vi "Initialize.vi"(8 "error in (no error)":errorcluster, 10 "DeviceName":string, 11 "FakePressureController in":refnum<class "PXIDigitizer.lvclass">) -> (0 "error out":errorcluster, 1 "new command(s)":string, 2 "DeviceName":string, 3 "FakePressureController out":refnum<class "PXIDigitizer.lvclass">)   [LabVIEW 2011, in "PXIDigitizer.lvclass"]
uses:
  PXIDigitizer.lvclass
  settings_TypDef.ctl
  numericVariable_TypeDef.ctl
  OnOffTypeDef.ctl
  channelenabled_TypDef.ctl
  coupling_Enum_TypDef.ctl
  impedance_Enum_TypDEf.ctl
  TriggerSettings_TypDef.ctl
  Polarity_TypDEf.ctl
  TVEvent_TypDef.ctl
  coupling_TypDef.ctl
  positive_negatice2_typDef.ctl
  TriggerSource_TypDef.ctl
  triggerwindowmode2_TypDef.ctl
  SignalFormat_TypDef.ctl
  mode_TypDef.ctl
  Trigger.DigitalSource_TypDEf.ctl
  horizontal_TypDef.ctl
  methodCluster_TypDEf.ctl
  method_TypDef.ctl
  LinkedChannelsCluster_TypDef.ctl
  channels_TypDef.ctl
  BaseDriver/BaseDriver.lvclass
  PXIDigitizer.lvclass/PXIDigitizer.ctl
panel:
  out "data":T1={"resourcename"="", "timeout"={"Value"=0.0, "Min"=0.0, "Max"=0.0, "StepSize"=0.0, "Tolerance"=0.0, "valueactual"=0.0}, "LocalSavingPath"=path "", "Save"=enum."off", "probeattenuation"={"Channel0"={"Value"=0.0, "Min"=0.0, "Max"=0.0, "StepSize"=0.0, "Tolerance"=0.0, "valueactual"=0.0}, "Channel1"={"Value"=0.0, "Min"=0.0, "Max"=0.0, "StepSize"=0.0, "Tolerance"=0.0, "valueactual"=0.0}, "Channel2"={"Value"=0.0, "Min"=0.0, "Max"=0.0, "StepSize"=0.0, "Tolerance"=0.0, "valueactual"=0.0}, "Channel3"={"Value"=0.0, "Min"=0.0, "Max"=0.0, "StepSize"=0.0, "Tolerance"=0.0, "valueactual"=0.0}, "Channel4"={"Value"=0.0, "Min"=0.0, "Max"=0.0, "StepSize"=0.0, "Tolerance"=0.0, "valueactual"=0.0}, "Channel5"={"Value"=0.0, "Min"=0.0, "Max"=0.0, "StepSize"=0.0, "Tolerance"=0.0, "valueactual"=0.0}, "Channel6"={"Value"=0.0, "Min"=0.0, "Max"=0.0, "StepSize"=0.0, "Tolerance"=0.0, "valueactual"=0.0}, "Channel7"={"Value"=0.0, "Min"=0.0, "Max"=0.0, "StepSize"=0.0, "Tolerance"=0.0, "valueactual"=0.0}}, "channelenabled"={"Channel0"=enum."off", "Channel1"=enum."off", "Channel2"=enum."off", "Channel3"=enum."off", "Channel4"=enum."off", "Channel5"=enum."off", "Channel6"=enum."off", "Channel7"=enum."off"}, "coupling"={"Channel0"=enum."AC", "Channel1"=enum."AC", "Channel2"=enum."AC", "Channel3"=enum."AC", "Channel4"=enum."AC", "Channel5"=enum."AC", "Channel6"=enum."AC", "Channel7"=enum."AC"}, "impedance"={"Channel0"=enum."1 mega ohm", "Channel1"=enum."1 mega ohm", "Channel2"=enum."1 mega ohm", "Channel3"=enum."1 mega ohm", "Channel4"=enum."1 mega ohm", "Channel5"=enum."1 mega ohm", "Channel6"=enum."1 mega ohm", "Channel7"=enum."1 mega ohm"}, "Trigger"={"DC Restore"=enum."off", "Polarity"=enum."Negative", "TV Event"=enum."Field 1", "Coupling"=enum."AC", "Slope"=enum."Negative", "AnalogSource"=enum."Channel 0", "Window Mode"=enum."Entering", "Low Level"=0.0, "High Level"=0.0, "Hysteresis"=0.0, "Delay"=0.0, "Holdoff"=0.0, "Signal Format"=enum."M-NTSC", "Mode"=enum."Immediate", "Line Number"=0, "DigitalSource"=enum."RTSI 0"}, "Horizontal"={"min sample rate"=10000000.0, "min record length"=1000, "actual record length"=1000, "actual sample rate"=10000000.0, "Enforce Realtime"=enum."off"}, "Names"={"Channel0"="", "Channel1"="", "Channel2"="", "Channel3"="", "Channel4"="", "Channel5"="", "Channel6"="", "Channel7"=""}, "verticalrange"={"Channel0"={"Value"=0.0, "Min"=0.0, "Max"=0.0, "StepSize"=0.0, "Tolerance"=0.0, "valueactual"=0.0}, "Channel1"={"Value"=0.0, "Min"=0.0, "Max"=0.0, "StepSize"=0.0, "Tolerance"=0.0, "valueactual"=0.0}, "Channel2"={"Value"=0.0, "Min"=0.0, "Max"=0.0, "StepSize"=0.0, "Tolerance"=0.0, "valueactual"=0.0}, "Channel3"={"Value"=0.0, "Min"=0.0, "Max"=0.0, "StepSize"=0.0, "Tolerance"=0.0, "valueactual"=0.0}, "Channel4"={"Value"=0.0, "Min"=0.0, "Max"=0.0, "StepSize"=0.0, "Tolerance"=0.0, "valueactual"=0.0}, "Channel5"={"Value"=0.0, "Min"=0.0, "Max"=0.0, "StepSize"=0.0, "Tolerance"=0.0, "valueactual"=0.0}, "Channel6"={"Value"=0.0, "Min"=0.0, "Max"=0.0, "StepSize"=0.0, "Tolerance"=0.0, "valueactual"=0.0}, "Channel7"={"Value"=0.0, "Min"=0.0, "Max"=0.0, "StepSize"=0.0, "Tolerance"=0.0, "valueactual"=0.0}}, "offset"={"Channel0"={"Value"=0.0, "Min"=0.0, "Max"=0.0, "StepSize"=0.0, "Tolerance"=0.0, "valueactual"=0.0}, "Channel1"={"Value"=0.0, "Min"=0.0, "Max"=0.0, "StepSize"=0.0, "Tolerance"=0.0, "valueactual"=0.0}, "Channel2"={"Value"=0.0, "Min"=0.0, "Max"=0.0, "StepSize"=0.0, "Tolerance"=0.0, "valueactual"=0.0}, "Channel3"={"Value"=0.0, "Min"=0.0, "Max"=0.0, "StepSize"=0.0, "Tolerance"=0.0, "valueactual"=0.0}, "Channel4"={"Value"=0.0, "Min"=0.0, "Max"=0.0, "StepSize"=0.0, "Tolerance"=0.0, "valueactual"=0.0}, "Channel5"={"Value"=0.0, "Min"=0.0, "Max"=0.0, "StepSize"=0.0, "Tolerance"=0.0, "valueactual"=0.0}, "Channel6"={"Value"=0.0, "Min"=0.0, "Max"=0.0, "StepSize"=0.0, "Tolerance"=0.0, "valueactual"=0.0}, "Channel7"={"Value"=0.0, "Min"=0.0, "Max"=0.0, "StepSize"=0.0, "Tolerance"=0.0, "valueactual"=0.0}}, "Number of channels"=0.0, "Method"={"Analysis1"=enum."max", "Analysis2"=enum."max", "Analysis3"=enum."max", "Analysis4"=enum."max", "Analysis5"=enum."max", "Analysis6"=enum."max", "Analysis7"=enum."max", "Analysis8"=enum."max", "Analysis9"=enum."max", "Analysis10"=enum."max"}, "LinkedChannel"={"Analysis1"=enum."Channel0", "Analysis2"=enum."Channel0", "Analysis3"=enum."Channel0", "Analysis4"=enum."Channel0", "Analysis5"=enum."Channel0", "Analysis6"=enum."Channel0", "Analysis7"=enum."Channel0", "Analysis8"=enum."Channel0", "Analysis9"=enum."Channel0", "Analysis10"=enum."Channel0"}} {"Horizontal"."actual sample rate" format="%.2p"; "Horizontal"."min sample rate" step=1000000.0 format="%.2p"; "Trigger"."Delay" format="%#_12e"; "Trigger"."Holdoff" format="%#_12e"}
  out "Settings.resourcename":string
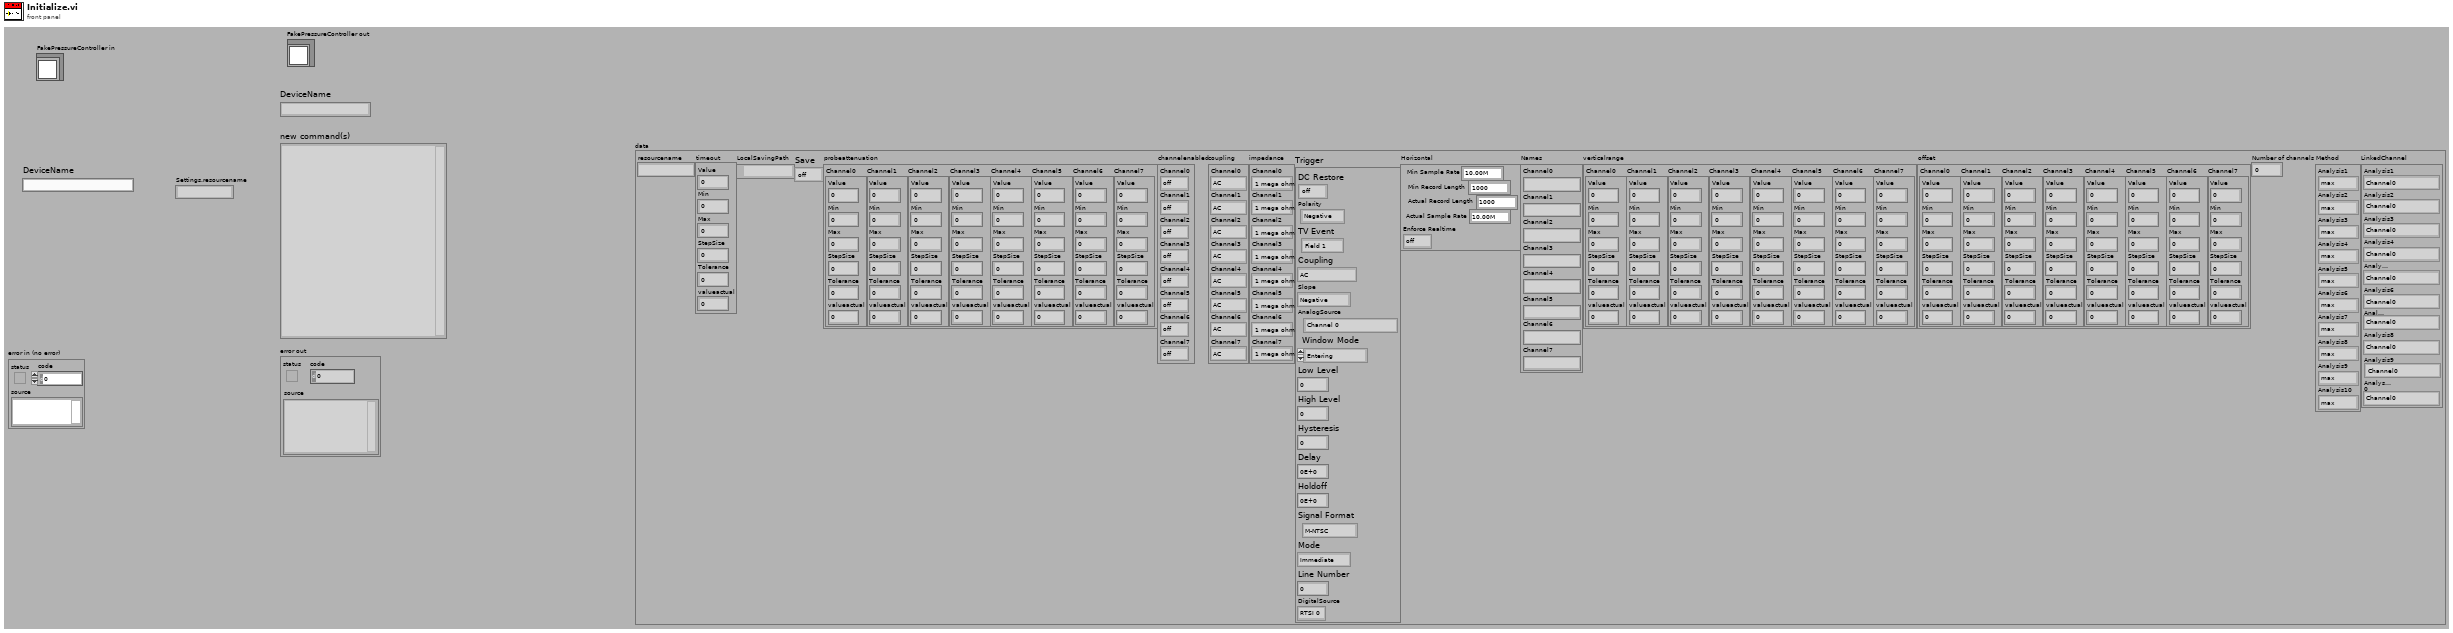
[diagram p1: front panel]
types:
  T1 = typedef "PXIDigitizer.lvclass/settings_TypDef.ctl" = cluster{"resourcename":string, "timeout":T2, "LocalSavingPath":path, "Save":T3, "probeattenuation":cluster{"Channel0":T2, "Channel1":T2, "Channel2":T2, "Channel3":T2, "Channel4":T2, "Channel5":T2, "Channel6":T2, "Channel7":T2}, "channelenabled":T4, "coupling":cluster{"Channel0":T5, "Channel1":T5, "Channel2":T5, "Channel3":T5, "Channel4":T5, "Channel5":T5, "Channel6":T5, "Channel7":T5}, "impedance":cluster{"Channel0":T6, "Channel1":T6, "Channel2":T6, "Channel3":T6, "Channel4":T6, "Channel5":T6, "Channel6":T6, "Channel7":T6}, "Trigger":T7, "Horizontal":T17, "Names":cluster{"Channel0":string, "Channel1":string, "Channel2":string, "Channel3":string, "Channel4":string, "Channel5":string, "Channel6":string, "Channel7":string}, "verticalrange":cluster{"Channel0":T2, "Channel1":T2, "Channel2":T2, "Channel3":T2, "Channel4":T2, "Channel5":T2, "Channel6":T2, "Channel7":T2}, "offset":cluster{"Channel0":T2, "Channel1":T2, "Channel2":T2, "Channel3":T2, "Channel4":T2, "Channel5":T2, "Channel6":T2, "Channel7":T2}, "Number of channels":dbl, "Method":T18, "LinkedChannel":T20}
  T2 = typedef "numericVariable_TypeDef.ctl" = cluster{"Value":dbl, "Min":dbl, "Max":dbl, "StepSize":dbl, "Tolerance":dbl, "valueactual":dbl}
  T3 = typedef "OnOffTypeDef.ctl" = enum16{"off", "on"}
  T4 = typedef "channelenabled_TypDef.ctl" = cluster{"Channel0":T3, "Channel1":T3, "Channel2":T3, "Channel3":T3, "Channel4":T3, "Channel5":T3, "Channel6":T3, "Channel7":T3}
  T5 = typedef "coupling_Enum_TypDef.ctl" = enum16{"AC", "DC", "Ground"}
  T6 = typedef "impedance_Enum_TypDEf.ctl" = enum16{"1 mega ohm", "<NA>", "50 ohms"}
  T7 = typedef "TriggerSettings_TypDef.ctl" = cluster{"DC Restore":T3, "Polarity":T8, "TV Event":T9, "Coupling":T10, "Slope":T11, "AnalogSource":T12, "Window Mode":T13, "Low Level":dbl, "High Level":dbl, "Hysteresis":dbl, "Delay":dbl, "Holdoff":dbl, "Signal Format":T14, "Mode":T15, "Line Number":i32, "DigitalSource":T16}
  T8 = typedef "Polarity_TypDEf.ctl" = enum16{"Negative", "Positive"}
  T9 = typedef "TVEvent_TypDef.ctl" = enum16{"Field 1", "Field 2", "Any Field", "Any Line", "Line Number"}
  T10 = typedef "coupling_TypDef.ctl" = enum16{"AC", "DC", "HF Reject", "LF Reject", "AC Plus HF Reject"}
  T11 = typedef "positive_negatice2_typDef.ctl" = enum16{"Positive", "Negative"}
  T12 = typedef "TriggerSource_TypDef.ctl" = enum16{"Channel 0", "Channel 1", "External TRIG"}
  T13 = typedef "triggerwindowmode2_TypDef.ctl" = enum16{"Entering", "Leaving"}
  T14 = typedef "SignalFormat_TypDef.ctl" = enum16{"M-NTSC", "B/G-PAL", "SECAM", "M-PAL", "480i/59.94 fps", "480i/60 fps", "480p/59.94 Fps", "480p/60 Fps", "576i/50 fps", "576p/50 Fps", "720p/50 Fps", "720p/59.94 Fps", "720p/60 Fps", "1080i/50 fps", "1080i/59.94 fps", "1080i/60 fps", "1080p/24 Fps"}
  T15 = typedef "mode_TypDef.ctl" = enum32{"Immediate", "Analog Edge", "Analog Window", "Analog Hysteresis", "Video", "Digital Edge"}
  T16 = typedef "Trigger.DigitalSource_TypDEf.ctl" = enum16{"RTSI 0", "RTSI 1", "RTSI 2", "RTSI 3", "RTSI 4", "RTSI 5", "RTSI 6", "PFI 0", "PFI 1", "PFI 2", "PXI Star Trigger"}
  T17 = typedef "horizontal_TypDef.ctl" = cluster{"min sample rate":dbl, "min record length":i32, "actual record length":i32, "actual sample rate":dbl, "Enforce Realtime":T3}
  T18 = typedef "methodCluster_TypDEf.ctl" = cluster{"Analysis1":T19, "Analysis2":T19, "Analysis3":T19, "Analysis4":T19, "Analysis5":T19, "Analysis6":T19, "Analysis7":T19, "Analysis8":T19, "Analysis9":T19, "Analysis10":T19}
  T19 = typedef "method_TypDef.ctl" = enum16{"n/a", "max", "min", "energy"}
  T20 = typedef "LinkedChannelsCluster_TypDef.ctl" = cluster{"Analysis1":T21, "Analysis2":T21, "Analysis3":T21, "Analysis4":T21, "Analysis5":T21, "Analysis6":T21, "Analysis7":T21, "Analysis8":T21, "Analysis9":T21, "Analysis10":T21}
  T21 = typedef "channels_TypDef.ctl" = enum16{"Channel0", "Channel1", "Channel2", "Channel3", "Channel4", "Channel5", "Channel6", "Channel7", "n/a"}
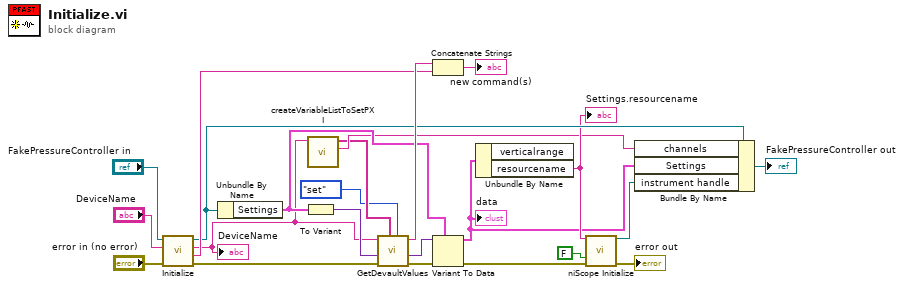
[diagram p0: block diagram]
diagram:
  n1 = call-parent "Initialize.vi"("error in (no error)"="error in (no error)", "DeviceName"="DeviceName", "BaseDriver in"="FakePressureController in") -> ("error out"=w10:errorcluster, "new command(s)"=w16:string, "DeviceName"=w4:string, "BaseDriver out"=w15:refnum<class "PXIDigitizer.lvclass">)  [unwired: 5 in]
  "DeviceName" <- w4
  n2 = Unbundle By Name(w15) -> ("Settings"=w17:T1)
  n3 = To Variant(anything=w17) -> (Variant=w18:variant)
  n4 = call "createVariableListToSetPXI.vi"("DeviceName"=w4) -> ("String"=w5:string, "Array"=w3:string[])  [unwired: 9 in]
  n5 = call "GetDevaultValues.vi"("set or DON'T set"=enum16{"set", "DON'T set"}."set", "set following Variables (empty = all avriables)"=w3, "error in (no error)"=w10, "variant"=w18, "Device Name"=w4) -> ("error out"=w9:errorcluster, "variant out"=w19:variant, "new command(s)"=w20:string)  [unwired: 4 in]
  n6 = Concatenate Strings(w20, w16) -> (→"new command(s)":string)
  n7 = Variant To Data(error in=w9, type=w17, Variant=w19) -> (data=w6:T1, error out=w12:errorcluster)
  "data" <- w6
  n8 = Unbundle By Name(w6) -> ("resourcename"=w11:string)  [unwired: 1 out]
  "Settings.resourcename" <- w11
  n9 = call "niScope Initialize.vi"("resource name"=w11, "reset device"=FALSE, "error in"=w12) -> ("instrument handle"=w8:refnum<k15>, "error out"=→"error out":errorcluster)  [unwired: 2 in, 9 out]
  n10 = Bundle By Name(cluster=w15, "channels"=w5, "Settings"=w6, "instrument handle"=w8) -> (→"FakePressureController out":refnum<class "PXIDigitizer.lvclass">)
